vi "Do.vi"(6 "Input":variant, 8 "error in":errorcluster, 9 "Self Enqueuer":refnum<class "Message Enqueuer.lvclass">, 10 "Series Enqueuer":refnum<class "Message Enqueuer.lvclass">, 11 "Sample PID Watervalve in":refnum<class "Sample PID Flow.lvclass">) -> (0 "error out":errorcluster, 3 "Sample PID Watervalve out":refnum<class "Sample PID Flow.lvclass">)   [LabVIEW 2023, in "Sample PID Flow.lvclass"]
uses:
  Sample PID Flow.lvclass
  <vilib>/ActorFramework/Message Enqueuer/Message Enqueuer.lvclass
  Task/ITask Actor/ITask Actor Messages/Do Msg/Do Msg.lvclass
  Task/Task Base/Task Base.lvclass/Task Base.ctl
  Series/ISeries Actor/ISeries Actor Messages/Point Data Updated Msg/Point Data Updated Msg.lvclass/Point Data Updated Msg.ctl
  <vilib>/ActorFramework/Message Enqueuer/Message Enqueuer.lvclass/Message Enqueuer.ctl
  <vilib>/ActorFramework/Message Enqueuer/Enqueue.vi
  Series/ISeries Actor/ISeries Actor Messages/Point Data Updated Msg/Point Data Updated Msg.lvclass
  <vilib>/Utility/LVClass/Get LV Class Name.vi
  <resource>/AFDebug/Generate Trace for Message.vi
  <vilib>/ActorFramework/Message Priority Queue/Priority Enqueue.vi
  <vilib>/addons/control/pid/pid.llb/PID (DBL).vi
  Sample PID Flow.lvclass/Sample PID Flow.ctl
  Task/Task Base/Task Base.lvclass
  <vilib>/addons/control/pid/NI_PID_pid.lvlib
  Measure and Stimulus Subsystems/Measure and Stimulus Subsystems.lvclass
  D:/git/HAL/HAL GOOP4/Task/Task Base/Task Base.lvclass
  D:/git/HAL/HAL GOOP4/Tests/Sample Tasks/Sample PID Flow/Sample PID Flow.lvclass
  C:/Program Files/National Instruments/LabVIEW 2023/vi.lib/ActorFramework/Message/Message.lvclass
  D:/git/HAL/HAL GOOP4/Task/ITask Actor/ITask Actor Messages/Do Msg/Do Msg.lvclass
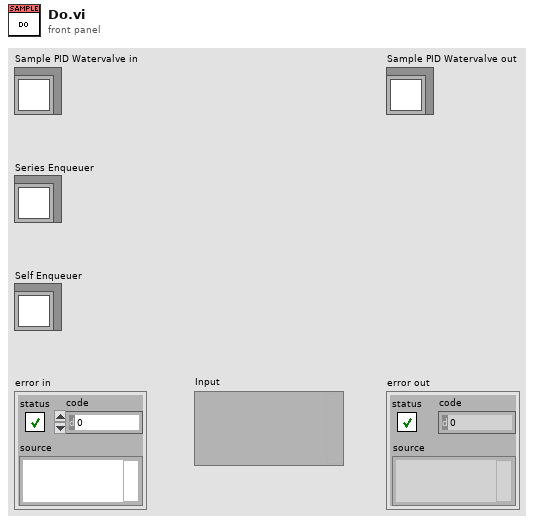
[diagram p1: front panel]
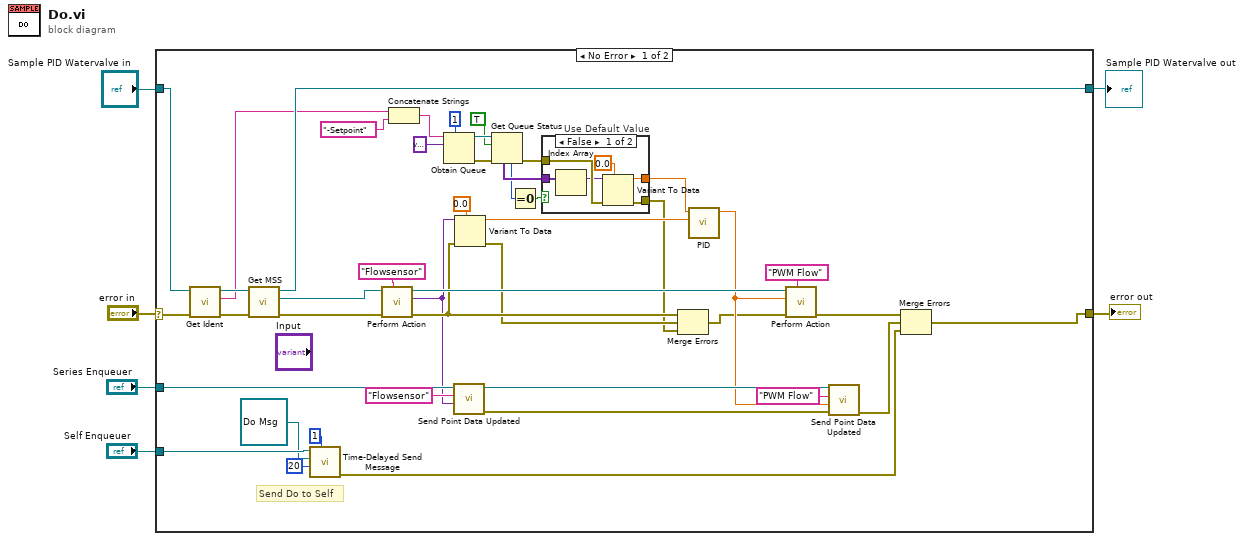
[diagram p0: block diagram]
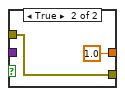
[diagram p2: hidden frame]
diagram:
  n1 = case shown="No Error" "error in" {
    selector: "error in" -> [w48 w60]
    tunnel: [w50 w60] -> w3
    tunnel: [w47 w59] -> w4
    tunnel: "Sample PID Watervalve in" -> [w16 w59]
    tunnel: "Series Enqueuer" -> [w49 _]
    tunnel: "Self Enqueuer" -> [w21 _]
    frame No Error {
      # "Send Do to Self"
      n2 = call "Get Ident.vi"("error in (no error)"=w48, "Task Base in"=w16) -> ("error out"=w17:errorcluster, "Ident"=w9:string, "Task Base out"=w15:refnum<class "Sample PID Flow.lvclass">)  [unwired: 7 in]
      n3 = call "Get MSS.vi"("error in (no error)"=w17, "Task Base in"=w15) -> ("error out"=w46:errorcluster, "MSS"=w45:refnum<class "Measure and Stimulus Subsystems.lvclass">, "Task Base out"=w47:refnum<class "Sample PID Flow.lvclass">)  [unwired: 7 in]
      n4 = call <vilib>:"Time-Delayed Send Message.vi"("# Copies (0 = infinite repeat)"=u32 1, "Milliseconds To Wait"=20, "Message"=refnum<class "Do Msg.lvclass"> refnum ("HAL GOOP4.lvlib:ITask Actor.lvlib:Do Msg.lvclass"), "Message Enqueuer"=w21) -> ("error out"=w8:errorcluster)  [unwired: 6 in, 1 out]
      n5 = call "Perform Action.vi"("Point Ident"="Flowsensor" ("Target Identifier"), "error in"=w46, "MSS in"=w45) -> ("error out"=w38:errorcluster, "Output"=w36:variant, "MSS out"=w39:refnum<class "Measure and Stimulus Subsystems.lvclass">)  [unwired: 6 in]
      n6 = Concatenate Strings(w9, "-Setpoint" ("string")) -> (w30:string)
      n7 = Obtain Queue(max queue size (-1, unlimited)=1, name (unnamed)=w30, element data type=variant) -> (queue out=w27:refnum<queue>, error out=w28:errorcluster)  [unwired: 2 in, 1 out]
      n8 = call "Send Point Data Updated.vi"("Data"=w36, "Point Ident"="Flowsensor" ("Name"), "Message Enqueuer"=w49) -> ("error out"=w32:errorcluster, "Message Enqueuer out"=w35:refnum<class "Message Enqueuer.lvclass">)  [unwired: 7 in]
      n9 = Variant To Data(error in=w38, type=0.0, Variant=w36) -> (data=w41:dbl, error out=w24:errorcluster)
      n10 = Get Queue Status(queue=w27, return elements? (F)=TRUE, error in (no error)=w28) -> (error out=w25:errorcluster, # elements in queue=w18:i32, elements=w20:variant[])  [unwired: 5 out]
      n11 = Equal To 0?(x=w18) -> (x = 0?=w19:bool)
      n12 = case "Use Default Value" shown="False" w19 {
        tunnel: w25 -> [w56 w57]
        tunnel: [w55 w57] -> w23
        tunnel: [w54 1.0] -> w22
        tunnel: w20 -> [w52 _]
        frame False {
          n13 = Index Array(array=w52) -> (element=w51:variant)  [unwired: 1 in]
          n14 = Variant To Data(error in=w56, type=0.0, Variant=w51) -> (data=w54:dbl, error out=w55:errorcluster)
        }
        frame True {
        }
      }
      n15 = Merge Errors(w38, w24, w23) -> (w26:errorcluster)
      n16 = call-poly <vilib>:"PID.vi"("process variable"=w41, "setpoint"=w22) -> ("output"=w33:dbl)  [unwired: 8 in, 1 out]
      n17 = call "Perform Action.vi"("Point Ident"="PWM Flow" ("Target Ident"), "error in"=w26, "Input"=w33, "MSS in"=w39) -> ("error out"=w40:errorcluster)  [unwired: 5 in, 2 out]
      n18 = call "Send Point Data Updated.vi"("error in (no error)"=w32, "Data"=w33, "Point Ident"="PWM Flow" ("Target Ident"), "Message Enqueuer"=w35) -> ("error out"=w7:errorcluster)  [unwired: 6 in, 1 out]
      n19 = Merge Errors(w40, w7, w8) -> (w50:errorcluster)
    }
    frame Error {
    }
  }
  "error out" <- w3
  "Sample PID Watervalve out" <- w4
